vi "Path flags.vi"() -> (4 "table_path()column_path":string, 6 "column_path()table_name":string, 8 "table_name()column_name":string, 10 "column_name()units":string, 15 "units()":string)   [LabVIEW 2019, in "LV-Data.PGSQL.lvclass"]
uses:
  LV-Data.PGSQL.lvclass
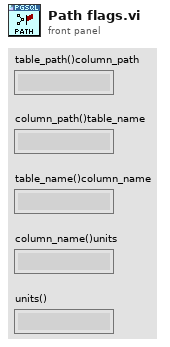
[diagram p1: front panel]
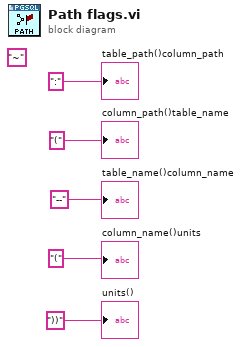
[diagram p0: block diagram]
diagram:
  (unwired) "~" ("table_path()column_path")
  "table_path()column_path" <- ":" ("table_path()column_path")
  "column_path()table_name" <- "(" ("column_path()table_name")
  "table_name()column_name" <- "--" ("table_name()column_name")
  "column_name()units" <- "(" ("column_name()units")
  "units()" <- "))" ("units()")
